vi "S4GUI.vi"(7 "Tab ObsEng":enum32{"Obs", "CCD modes", "Eng"}(tab)) -> ()   [LabVIEW 2018] (continued)
        n4535 = call "Write WPSEL.vi"("error in (no error)"=w10848, "Opt_Selector.lvclass"=w10850, "Instrument in"=w10849) -> ("error out"=w10845:errorcluster, "Instrument out"=w10847:refnum<class "Instrument.lvclass">)  [unwired: 7 in]
        n4536 = call "Write Instrument.lvclass.vi"("error in (no error)"=w10845, "Instrument.lvclass"=w10847, "S4ACS_GUI in"=w10846) -> ("error out"=w10844:errorcluster, "S4ACS_GUI out"=w10843:refnum<class "S4GUI.lvclass">)  [unwired: 7 in]
      }
      event "GMIR_target": Value Change {
        n4537 = event-data() -> ("NewVal"=w10872:dbl)  [unwired: 1 in, 3 out]
        n4538 = call "Read Instrument.lvclass.vi"("error in (no error)"=w10876, "S4ACS_GUI in"=w10877) -> ("error out"=w10874:errorcluster, "Instrument.lvclass"=w10875:refnum<class "Instrument.lvclass">, "S4ACS_GUI out"=w10866:refnum<class "S4GUI.lvclass">)  [unwired: 7 in]
        n4539 = call "Read GMIR.vi"("error in (no error)"=w10874, "Instrument in"=w10875) -> ("error out"=w10871:errorcluster, "Opt_Continuous.lvclass"=w10873:refnum<class "Opt_Continuous.lvclass">, "Instrument out"=w10869:refnum<class "Instrument.lvclass">)  [unwired: 7 in]
        n4540 = call "Write target.vi"("error in (no error)"=w10871, "target"=w10872, "Optics in"=w10873) -> ("error out"=w10868:errorcluster, "Optics out"=w10870:refnum<class "Opt_Continuous.lvclass">)  [unwired: 7 in]
        n4541 = call "Write GMIR.vi"("error in (no error)"=w10868, "Opt_Continuous.lvclass"=w10870, "Instrument in"=w10869) -> ("error out"=w10865:errorcluster, "Instrument out"=w10867:refnum<class "Instrument.lvclass">)  [unwired: 7 in]
        n4542 = call "Write Instrument.lvclass.vi"("error in (no error)"=w10865, "Instrument.lvclass"=w10867, "S4ACS_GUI in"=w10866) -> ("error out"=w10864:errorcluster, "S4ACS_GUI out"=w10863:refnum<class "S4GUI.lvclass">)  [unwired: 7 in]
      }
      event "GMIR_set": Value Change {
        n4543 = event-data() -> ()  [unwired: 1 in, 4 out]
        n4544 = call "Read Instrument.lvclass.vi"("error in (no error)"=w10896, "S4ACS_GUI in"=w10897) -> ("error out"=w10894:errorcluster, "Instrument.lvclass"=w10895:refnum<class "Instrument.lvclass">, "S4ACS_GUI out"=w10883:refnum<class "S4GUI.lvclass">)  [unwired: 7 in]
        n4545 = call "Read GMIR.vi"("error in (no error)"=w10894, "Instrument in"=w10895) -> ("error out"=w10891:errorcluster, "Opt_Continuous.lvclass"=w10893:refnum<class "Opt_Continuous.lvclass">, "Instrument out"=w10885:refnum<class "Instrument.lvclass">)  [unwired: 7 in]
        n4546 = call-dynamic "Read State Machine.vi"("error in (no error)"=w10891, "Device in"=w10893) -> ("error out"=w10890:errorcluster, "State Machine.lvclass"=w10881:refnum<class "State Machine.lvclass">, "Device out"=w10887:refnum<class "Opt_Continuous.lvclass">)  [unwired: 7 in]
        n4547 = call "Next State.vi"("error in (no error)"=w10890, "New_State"=1, "State Machine in"=w10881) -> ("error out"=w10889:errorcluster, "State Machine out"=w10888:refnum<class "State Machine.lvclass">)  [unwired: 7 in]
        n4548 = call-dynamic "Write State Machine.vi"("error in (no error)"=w10889, "State Machine.lvclass"=w10888, "Device in"=w10887) -> ("error out"=w10884:errorcluster, "Device out"=w10886:refnum<class "Opt_Continuous.lvclass">)  [unwired: 7 in]
        n4549 = call "Write GMIR.vi"("error in (no error)"=w10884, "Opt_Continuous.lvclass"=w10886, "Instrument in"=w10885) -> ("error out"=w10878:errorcluster, "Instrument out"=w10879:refnum<class "Instrument.lvclass">)  [unwired: 7 in]
        n4550 = call "Write Instrument.lvclass.vi"("error in (no error)"=w10878, "Instrument.lvclass"=w10879, "S4ACS_GUI in"=w10883) -> ("error out"=w10882:errorcluster, "S4ACS_GUI out"=w10880:refnum<class "S4GUI.lvclass">)  [unwired: 7 in]
      }
      event "GMIR_stop": Value Change {
        n4551 = event-data() -> ()  [unwired: 1 in, 4 out]
        n4552 = call "Read Instrument.lvclass.vi"("error in (no error)"=w10916, "S4ACS_GUI in"=w10917) -> ("error out"=w10914:errorcluster, "Instrument.lvclass"=w10915:refnum<class "Instrument.lvclass">, "S4ACS_GUI out"=w10901:refnum<class "S4GUI.lvclass">)  [unwired: 7 in]
        n4553 = call "Read GMIR.vi"("error in (no error)"=w10914, "Instrument in"=w10915) -> ("error out"=w10910:errorcluster, "Opt_Continuous.lvclass"=w10913:refnum<class "Opt_Continuous.lvclass">, "Instrument out"=w10904:refnum<class "Instrument.lvclass">)  [unwired: 7 in]
        n4554 = call-dynamic "Read State Machine.vi"("error in (no error)"=w10910, "Device in"=w10913) -> ("error out"=w10909:errorcluster, "State Machine.lvclass"=w10912:refnum<class "State Machine.lvclass">, "Device out"=w10906:refnum<class "Opt_Continuous.lvclass">)  [unwired: 7 in]
        n4555 = call "Next State.vi"("error in (no error)"=w10909, "New_State"=10, "State Machine in"=w10912) -> ("error out"=w10908:errorcluster, "State Machine out"=w10907:refnum<class "State Machine.lvclass">)  [unwired: 7 in]
        n4556 = call-dynamic "Write State Machine.vi"("error in (no error)"=w10908, "State Machine.lvclass"=w10907, "Device in"=w10906) -> ("error out"=w10903:errorcluster, "Device out"=w10905:refnum<class "Opt_Continuous.lvclass">)  [unwired: 7 in]
        n4557 = call "Write GMIR.vi"("error in (no error)"=w10903, "Opt_Continuous.lvclass"=w10905, "Instrument in"=w10904) -> ("error out"=w10900:errorcluster, "Instrument out"=w10902:refnum<class "Instrument.lvclass">)  [unwired: 7 in]
        n4558 = call "Write Instrument.lvclass.vi"("error in (no error)"=w10900, "Instrument.lvclass"=w10902, "S4ACS_GUI in"=w10901) -> ("error out"=w10899:errorcluster, "S4ACS_GUI out"=w10898:refnum<class "S4GUI.lvclass">)  [unwired: 7 in]
      }
      event "GMIR_init": Value Change {
        n4559 = event-data() -> ()  [unwired: 1 in, 4 out]
        n4560 = call "Read Instrument.lvclass.vi"("error in (no error)"=w10936, "S4ACS_GUI in"=w10937) -> ("error out"=w10934:errorcluster, "Instrument.lvclass"=w10935:refnum<class "Instrument.lvclass">, "S4ACS_GUI out"=w10921:refnum<class "S4GUI.lvclass">)  [unwired: 7 in]
        n4561 = call "Read GMIR.vi"("error in (no error)"=w10934, "Instrument in"=w10935) -> ("error out"=w10930:errorcluster, "Opt_Continuous.lvclass"=w10933:refnum<class "Opt_Continuous.lvclass">, "Instrument out"=w10924:refnum<class "Instrument.lvclass">)  [unwired: 7 in]
        n4562 = call-dynamic "Read State Machine.vi"("error in (no error)"=w10930, "Device in"=w10933) -> ("error out"=w10929:errorcluster, "State Machine.lvclass"=w10932:refnum<class "State Machine.lvclass">, "Device out"=w10926:refnum<class "Opt_Continuous.lvclass">)  [unwired: 7 in]
        n4563 = call "Next State.vi"("error in (no error)"=w10929, "New_State"=30, "State Machine in"=w10932) -> ("error out"=w10928:errorcluster, "State Machine out"=w10927:refnum<class "State Machine.lvclass">)  [unwired: 7 in]
        n4564 = call-dynamic "Write State Machine.vi"("error in (no error)"=w10928, "State Machine.lvclass"=w10927, "Device in"=w10926) -> ("error out"=w10923:errorcluster, "Device out"=w10925:refnum<class "Opt_Continuous.lvclass">)  [unwired: 7 in]
        n4565 = call "Write GMIR.vi"("error in (no error)"=w10923, "Opt_Continuous.lvclass"=w10925, "Instrument in"=w10924) -> ("error out"=w10920:errorcluster, "Instrument out"=w10922:refnum<class "Instrument.lvclass">)  [unwired: 7 in]
        n4566 = call "Write Instrument.lvclass.vi"("error in (no error)"=w10920, "Instrument.lvclass"=w10922, "S4ACS_GUI in"=w10921) -> ("error out"=w10919:errorcluster, "S4ACS_GUI out"=w10918:refnum<class "S4GUI.lvclass">)  [unwired: 7 in]
      }
      event "GFOC_target": Value Change {
        n4567 = event-data() -> ("NewVal"=w10947:dbl)  [unwired: 1 in, 3 out]
        n4568 = call "Read Instrument.lvclass.vi"("error in (no error)"=w10951, "S4ACS_GUI in"=w10952) -> ("error out"=w10949:errorcluster, "Instrument.lvclass"=w10950:refnum<class "Instrument.lvclass">, "S4ACS_GUI out"=w10941:refnum<class "S4GUI.lvclass">)  [unwired: 7 in]
        n4569 = call "Read GFOC.vi"("error in (no error)"=w10949, "Instrument in"=w10950) -> ("error out"=w10946:errorcluster, "Opt_Continuous.lvclass"=w10948:refnum<class "Opt_Continuous.lvclass">, "Instrument out"=w10944:refnum<class "Instrument.lvclass">)  [unwired: 7 in]
        n4570 = call "Write target.vi"("error in (no error)"=w10946, "target"=w10947, "Optics in"=w10948) -> ("error out"=w10943:errorcluster, "Optics out"=w10945:refnum<class "Opt_Continuous.lvclass">)  [unwired: 7 in]
        n4571 = call "Write GFOC.vi"("error in (no error)"=w10943, "Opt_Continuous.lvclass"=w10945, "Instrument in"=w10944) -> ("error out"=w10940:errorcluster, "Instrument out"=w10942:refnum<class "Instrument.lvclass">)  [unwired: 7 in]
        n4572 = call "Write Instrument.lvclass.vi"("error in (no error)"=w10940, "Instrument.lvclass"=w10942, "S4ACS_GUI in"=w10941) -> ("error out"=w10939:errorcluster, "S4ACS_GUI out"=w10938:refnum<class "S4GUI.lvclass">)  [unwired: 7 in]
      }
      event "GFOC_set": Value Change {
        n4573 = event-data() -> ()  [unwired: 1 in, 4 out]
        n4574 = call "Read Instrument.lvclass.vi"("error in (no error)"=w10971, "S4ACS_GUI in"=w10972) -> ("error out"=w10969:errorcluster, "Instrument.lvclass"=w10970:refnum<class "Instrument.lvclass">, "S4ACS_GUI out"=w10957:refnum<class "S4GUI.lvclass">)  [unwired: 7 in]
        n4575 = call "Read GFOC.vi"("error in (no error)"=w10969, "Instrument in"=w10970) -> ("error out"=w10966:errorcluster, "Opt_Continuous.lvclass"=w10968:refnum<class "Opt_Continuous.lvclass">, "Instrument out"=w10960:refnum<class "Instrument.lvclass">)  [unwired: 7 in]
        n4576 = call-dynamic "Read State Machine.vi"("error in (no error)"=w10966, "Device in"=w10968) -> ("error out"=w10965:errorcluster, "State Machine.lvclass"=w10954:refnum<class "State Machine.lvclass">, "Device out"=w10962:refnum<class "Opt_Continuous.lvclass">)  [unwired: 7 in]
        n4577 = call "Next State.vi"("error in (no error)"=w10965, "New_State"=1, "State Machine in"=w10954) -> ("error out"=w10964:errorcluster, "State Machine out"=w10963:refnum<class "State Machine.lvclass">)  [unwired: 7 in]
        n4578 = call-dynamic "Write State Machine.vi"("error in (no error)"=w10964, "State Machine.lvclass"=w10963, "Device in"=w10962) -> ("error out"=w10959:errorcluster, "Device out"=w10961:refnum<class "Opt_Continuous.lvclass">)  [unwired: 7 in]
        n4579 = call "Write GFOC.vi"("error in (no error)"=w10959, "Opt_Continuous.lvclass"=w10961, "Instrument in"=w10960) -> ("error out"=w10956:errorcluster, "Instrument out"=w10958:refnum<class "Instrument.lvclass">)  [unwired: 7 in]
        n4580 = call "Write Instrument.lvclass.vi"("error in (no error)"=w10956, "Instrument.lvclass"=w10958, "S4ACS_GUI in"=w10957) -> ("error out"=w10955:errorcluster, "S4ACS_GUI out"=w10953:refnum<class "S4GUI.lvclass">)  [unwired: 7 in]
      }
      event "GFOC_stop": Value Change {
        n4581 = event-data() -> ()  [unwired: 1 in, 4 out]
        n4582 = call "Read Instrument.lvclass.vi"("error in (no error)"=w10991, "S4ACS_GUI in"=w10992) -> ("error out"=w10989:errorcluster, "Instrument.lvclass"=w10990:refnum<class "Instrument.lvclass">, "S4ACS_GUI out"=w10976:refnum<class "S4GUI.lvclass">)  [unwired: 7 in]
        n4583 = call "Read GFOC.vi"("error in (no error)"=w10989, "Instrument in"=w10990) -> ("error out"=w10985:errorcluster, "Opt_Continuous.lvclass"=w10988:refnum<class "Opt_Continuous.lvclass">, "Instrument out"=w10979:refnum<class "Instrument.lvclass">)  [unwired: 7 in]
        n4584 = call-dynamic "Read State Machine.vi"("error in (no error)"=w10985, "Device in"=w10988) -> ("error out"=w10984:errorcluster, "State Machine.lvclass"=w10987:refnum<class "State Machine.lvclass">, "Device out"=w10981:refnum<class "Opt_Continuous.lvclass">)  [unwired: 7 in]
        n4585 = call "Next State.vi"("error in (no error)"=w10984, "New_State"=10, "State Machine in"=w10987) -> ("error out"=w10983:errorcluster, "State Machine out"=w10982:refnum<class "State Machine.lvclass">)  [unwired: 7 in]
        n4586 = call-dynamic "Write State Machine.vi"("error in (no error)"=w10983, "State Machine.lvclass"=w10982, "Device in"=w10981) -> ("error out"=w10978:errorcluster, "Device out"=w10980:refnum<class "Opt_Continuous.lvclass">)  [unwired: 7 in]
        n4587 = call "Write GFOC.vi"("error in (no error)"=w10978, "Opt_Continuous.lvclass"=w10980, "Instrument in"=w10979) -> ("error out"=w10975:errorcluster, "Instrument out"=w10977:refnum<class "Instrument.lvclass">)  [unwired: 7 in]
        n4588 = call "Write Instrument.lvclass.vi"("error in (no error)"=w10975, "Instrument.lvclass"=w10977, "S4ACS_GUI in"=w10976) -> ("error out"=w10974:errorcluster, "S4ACS_GUI out"=w10973:refnum<class "S4GUI.lvclass">)  [unwired: 7 in]
      }
      event "GFOC_init": Value Change {
        n4589 = event-data() -> ()  [unwired: 1 in, 4 out]
        n4590 = call "Read Instrument.lvclass.vi"("error in (no error)"=w11011, "S4ACS_GUI in"=w11012) -> ("error out"=w11009:errorcluster, "Instrument.lvclass"=w11010:refnum<class "Instrument.lvclass">, "S4ACS_GUI out"=w10996:refnum<class "S4GUI.lvclass">)  [unwired: 7 in]
        n4591 = call "Read GFOC.vi"("error in (no error)"=w11009, "Instrument in"=w11010) -> ("error out"=w11005:errorcluster, "Opt_Continuous.lvclass"=w11008:refnum<class "Opt_Continuous.lvclass">, "Instrument out"=w10999:refnum<class "Instrument.lvclass">)  [unwired: 7 in]
        n4592 = call-dynamic "Read State Machine.vi"("error in (no error)"=w11005, "Device in"=w11008) -> ("error out"=w11004:errorcluster, "State Machine.lvclass"=w11007:refnum<class "State Machine.lvclass">, "Device out"=w11001:refnum<class "Opt_Continuous.lvclass">)  [unwired: 7 in]
        n4593 = call "Next State.vi"("error in (no error)"=w11004, "New_State"=30, "State Machine in"=w11007) -> ("error out"=w11003:errorcluster, "State Machine out"=w11002:refnum<class "State Machine.lvclass">)  [unwired: 7 in]
        n4594 = call-dynamic "Write State Machine.vi"("error in (no error)"=w11003, "State Machine.lvclass"=w11002, "Device in"=w11001) -> ("error out"=w10998:errorcluster, "Device out"=w11000:refnum<class "Opt_Continuous.lvclass">)  [unwired: 7 in]
        n4595 = call "Write GFOC.vi"("error in (no error)"=w10998, "Opt_Continuous.lvclass"=w11000, "Instrument in"=w10999) -> ("error out"=w10995:errorcluster, "Instrument out"=w10997:refnum<class "Instrument.lvclass">)  [unwired: 7 in]
        n4596 = call "Write Instrument.lvclass.vi"("error in (no error)"=w10995, "Instrument.lvclass"=w10997, "S4ACS_GUI in"=w10996) -> ("error out"=w10994:errorcluster, "S4ACS_GUI out"=w10993:refnum<class "S4GUI.lvclass">)  [unwired: 7 in]
      }
      event "CALW_target": Value Change {
        n4597 = event-data() -> ("NewVal"=w11022:dbl)  [unwired: 1 in, 3 out]
        n4598 = call "Read Instrument.lvclass.vi"("error in (no error)"=w11026, "S4ACS_GUI in"=w11027) -> ("error out"=w11024:errorcluster, "Instrument.lvclass"=w11025:refnum<class "Instrument.lvclass">, "S4ACS_GUI out"=w11016:refnum<class "S4GUI.lvclass">)  [unwired: 7 in]
        n4599 = call "Read CALW.vi"("error in (no error)"=w11024, "Instrument in"=w11025) -> ("error out"=w11021:errorcluster, "Opt_Selector.lvclass"=w11023:refnum<class "Opt_Selector.lvclass">, "Instrument out"=w11019:refnum<class "Instrument.lvclass">)  [unwired: 7 in]
        n4600 = call "Write target.vi"("error in (no error)"=w11021, "target"=w11022, "Optics in"=w11023) -> ("error out"=w11018:errorcluster, "Optics out"=w11020:refnum<class "Opt_Selector.lvclass">)  [unwired: 7 in]
        n4601 = call "Write CALW.vi"("error in (no error)"=w11018, "Opt_Selector.lvclass"=w11020, "Instrument in"=w11019) -> ("error out"=w11015:errorcluster, "Instrument out"=w11017:refnum<class "Instrument.lvclass">)  [unwired: 7 in]
        n4602 = call "Write Instrument.lvclass.vi"("error in (no error)"=w11015, "Instrument.lvclass"=w11017, "S4ACS_GUI in"=w11016) -> ("error out"=w11014:errorcluster, "S4ACS_GUI out"=w11013:refnum<class "S4GUI.lvclass">)  [unwired: 7 in]
      }
      event "CALW_set": Value Change {
        n4603 = event-data() -> ()  [unwired: 1 in, 4 out]
        n4604 = call "Read Instrument.lvclass.vi"("error in (no error)"=w11046, "S4ACS_GUI in"=w11047) -> ("error out"=w11044:errorcluster, "Instrument.lvclass"=w11045:refnum<class "Instrument.lvclass">, "S4ACS_GUI out"=w11032:refnum<class "S4GUI.lvclass">)  [unwired: 7 in]
        n4605 = call "Read CALW.vi"("error in (no error)"=w11044, "Instrument in"=w11045) -> ("error out"=w11041:errorcluster, "Opt_Selector.lvclass"=w11043:refnum<class "Opt_Selector.lvclass">, "Instrument out"=w11035:refnum<class "Instrument.lvclass">)  [unwired: 7 in]
        n4606 = call-dynamic "Read State Machine.vi"("error in (no error)"=w11041, "Device in"=w11043) -> ("error out"=w11040:errorcluster, "State Machine.lvclass"=w11029:refnum<class "State Machine.lvclass">, "Device out"=w11037:refnum<class "Opt_Selector.lvclass">)  [unwired: 7 in]
        n4607 = call "Next State.vi"("error in (no error)"=w11040, "New_State"=1, "State Machine in"=w11029) -> ("error out"=w11039:errorcluster, "State Machine out"=w11038:refnum<class "State Machine.lvclass">)  [unwired: 7 in]
        n4608 = call-dynamic "Write State Machine.vi"("error in (no error)"=w11039, "State Machine.lvclass"=w11038, "Device in"=w11037) -> ("error out"=w11034:errorcluster, "Device out"=w11036:refnum<class "Opt_Selector.lvclass">)  [unwired: 7 in]
        n4609 = call "Write CALW.vi"("error in (no error)"=w11034, "Opt_Selector.lvclass"=w11036, "Instrument in"=w11035) -> ("error out"=w11031:errorcluster, "Instrument out"=w11033:refnum<class "Instrument.lvclass">)  [unwired: 7 in]
        n4610 = call "Write Instrument.lvclass.vi"("error in (no error)"=w11031, "Instrument.lvclass"=w11033, "S4ACS_GUI in"=w11032) -> ("error out"=w11030:errorcluster, "S4ACS_GUI out"=w11028:refnum<class "S4GUI.lvclass">)  [unwired: 7 in]
      }
      event "CALW_stop": Value Change {
        n4611 = event-data() -> ()  [unwired: 1 in, 4 out]
        n4612 = call "Read Instrument.lvclass.vi"("error in (no error)"=w11066, "S4ACS_GUI in"=w11067) -> ("error out"=w11064:errorcluster, "Instrument.lvclass"=w11065:refnum<class "Instrument.lvclass">, "S4ACS_GUI out"=w11051:refnum<class "S4GUI.lvclass">)  [unwired: 7 in]
        n4613 = call "Read CALW.vi"("error in (no error)"=w11064, "Instrument in"=w11065) -> ("error out"=w11060:errorcluster, "Opt_Selector.lvclass"=w11063:refnum<class "Opt_Selector.lvclass">, "Instrument out"=w11054:refnum<class "Instrument.lvclass">)  [unwired: 7 in]
        n4614 = call-dynamic "Read State Machine.vi"("error in (no error)"=w11060, "Device in"=w11063) -> ("error out"=w11059:errorcluster, "State Machine.lvclass"=w11062:refnum<class "State Machine.lvclass">, "Device out"=w11056:refnum<class "Opt_Selector.lvclass">)  [unwired: 7 in]
        n4615 = call "Next State.vi"("error in (no error)"=w11059, "New_State"=10, "State Machine in"=w11062) -> ("error out"=w11058:errorcluster, "State Machine out"=w11057:refnum<class "State Machine.lvclass">)  [unwired: 7 in]
        n4616 = call-dynamic "Write State Machine.vi"("error in (no error)"=w11058, "State Machine.lvclass"=w11057, "Device in"=w11056) -> ("error out"=w11053:errorcluster, "Device out"=w11055:refnum<class "Opt_Selector.lvclass">)  [unwired: 7 in]
        n4617 = call "Write CALW.vi"("error in (no error)"=w11053, "Opt_Selector.lvclass"=w11055, "Instrument in"=w11054) -> ("error out"=w11050:errorcluster, "Instrument out"=w11052:refnum<class "Instrument.lvclass">)  [unwired: 7 in]
        n4618 = call "Write Instrument.lvclass.vi"("error in (no error)"=w11050, "Instrument.lvclass"=w11052, "S4ACS_GUI in"=w11051) -> ("error out"=w11049:errorcluster, "S4ACS_GUI out"=w11048:refnum<class "S4GUI.lvclass">)  [unwired: 7 in]
      }
      event "CALW_init": Value Change {
        n4619 = event-data() -> ()  [unwired: 1 in, 4 out]
        n4620 = call "Read Instrument.lvclass.vi"("error in (no error)"=w11086, "S4ACS_GUI in"=w11087) -> ("error out"=w11084:errorcluster, "Instrument.lvclass"=w11085:refnum<class "Instrument.lvclass">, "S4ACS_GUI out"=w11071:refnum<class "S4GUI.lvclass">)  [unwired: 7 in]
        n4621 = call "Read CALW.vi"("error in (no error)"=w11084, "Instrument in"=w11085) -> ("error out"=w11080:errorcluster, "Opt_Selector.lvclass"=w11083:refnum<class "Opt_Selector.lvclass">, "Instrument out"=w11074:refnum<class "Instrument.lvclass">)  [unwired: 7 in]
        n4622 = call-dynamic "Read State Machine.vi"("error in (no error)"=w11080, "Device in"=w11083) -> ("error out"=w11079:errorcluster, "State Machine.lvclass"=w11082:refnum<class "State Machine.lvclass">, "Device out"=w11076:refnum<class "Opt_Selector.lvclass">)  [unwired: 7 in]
        n4623 = call "Next State.vi"("error in (no error)"=w11079, "New_State"=30, "State Machine in"=w11082) -> ("error out"=w11078:errorcluster, "State Machine out"=w11077:refnum<class "State Machine.lvclass">)  [unwired: 7 in]
        n4624 = call-dynamic "Write State Machine.vi"("error in (no error)"=w11078, "State Machine.lvclass"=w11077, "Device in"=w11076) -> ("error out"=w11073:errorcluster, "Device out"=w11075:refnum<class "Opt_Selector.lvclass">)  [unwired: 7 in]
        n4625 = call "Write CALW.vi"("error in (no error)"=w11073, "Opt_Selector.lvclass"=w11075, "Instrument in"=w11074) -> ("error out"=w11070:errorcluster, "Instrument out"=w11072:refnum<class "Instrument.lvclass">)  [unwired: 7 in]
        n4626 = call "Write Instrument.lvclass.vi"("error in (no error)"=w11070, "Instrument.lvclass"=w11072, "S4ACS_GUI in"=w11071) -> ("error out"=w11069:errorcluster, "S4ACS_GUI out"=w11068:refnum<class "S4GUI.lvclass">)  [unwired: 7 in]
      }
      event "ASEL_target": Value Change {
        n4627 = event-data() -> ("NewVal"=w11097:dbl)  [unwired: 1 in, 3 out]
        n4628 = call "Read Instrument.lvclass.vi"("error in (no error)"=w11101, "S4ACS_GUI in"=w11102) -> ("error out"=w11099:errorcluster, "Instrument.lvclass"=w11100:refnum<class "Instrument.lvclass">, "S4ACS_GUI out"=w11091:refnum<class "S4GUI.lvclass">)  [unwired: 7 in]
        n4629 = call "Read ASEL.vi"("error in (no error)"=w11099, "Instrument in"=w11100) -> ("error out"=w11096:errorcluster, "Opt_Selector.lvclass"=w11098:refnum<class "Opt_Selector.lvclass">, "Instrument out"=w11094:refnum<class "Instrument.lvclass">)  [unwired: 7 in]
        n4630 = call "Write target.vi"("error in (no error)"=w11096, "target"=w11097, "Optics in"=w11098) -> ("error out"=w11093:errorcluster, "Optics out"=w11095:refnum<class "Opt_Selector.lvclass">)  [unwired: 7 in]
        n4631 = call "Write ASEL.vi"("error in (no error)"=w11093, "Opt_Selector.lvclass"=w11095, "Instrument in"=w11094) -> ("error out"=w11090:errorcluster, "Instrument out"=w11092:refnum<class "Instrument.lvclass">)  [unwired: 7 in]
        n4632 = call "Write Instrument.lvclass.vi"("error in (no error)"=w11090, "Instrument.lvclass"=w11092, "S4ACS_GUI in"=w11091) -> ("error out"=w11089:errorcluster, "S4ACS_GUI out"=w11088:refnum<class "S4GUI.lvclass">)  [unwired: 7 in]
      }
      event "ASEL_set": Value Change {
        n4633 = event-data() -> ()  [unwired: 1 in, 4 out]
        n4634 = call "Read Instrument.lvclass.vi"("error in (no error)"=w11121, "S4ACS_GUI in"=w11122) -> ("error out"=w11119:errorcluster, "Instrument.lvclass"=w11120:refnum<class "Instrument.lvclass">, "S4ACS_GUI out"=w11107:refnum<class "S4GUI.lvclass">)  [unwired: 7 in]
        n4635 = call "Read ASEL.vi"("error in (no error)"=w11119, "Instrument in"=w11120) -> ("error out"=w11116:errorcluster, "Opt_Selector.lvclass"=w11118:refnum<class "Opt_Selector.lvclass">, "Instrument out"=w11110:refnum<class "Instrument.lvclass">)  [unwired: 7 in]
        n4636 = call-dynamic "Read State Machine.vi"("error in (no error)"=w11116, "Device in"=w11118) -> ("error out"=w11115:errorcluster, "State Machine.lvclass"=w11104:refnum<class "State Machine.lvclass">, "Device out"=w11112:refnum<class "Opt_Selector.lvclass">)  [unwired: 7 in]
        n4637 = call "Next State.vi"("error in (no error)"=w11115, "New_State"=1, "State Machine in"=w11104) -> ("error out"=w11114:errorcluster, "State Machine out"=w11113:refnum<class "State Machine.lvclass">)  [unwired: 7 in]
        n4638 = call-dynamic "Write State Machine.vi"("error in (no error)"=w11114, "State Machine.lvclass"=w11113, "Device in"=w11112) -> ("error out"=w11109:errorcluster, "Device out"=w11111:refnum<class "Opt_Selector.lvclass">)  [unwired: 7 in]
        n4639 = call "Write ASEL.vi"("error in (no error)"=w11109, "Opt_Selector.lvclass"=w11111, "Instrument in"=w11110) -> ("error out"=w11106:errorcluster, "Instrument out"=w11108:refnum<class "Instrument.lvclass">)  [unwired: 7 in]
        n4640 = call "Write Instrument.lvclass.vi"("error in (no error)"=w11106, "Instrument.lvclass"=w11108, "S4ACS_GUI in"=w11107) -> ("error out"=w11105:errorcluster, "S4ACS_GUI out"=w11103:refnum<class "S4GUI.lvclass">)  [unwired: 7 in]
      }
      event "ASEL_stop": Value Change {
        n4641 = event-data() -> ()  [unwired: 1 in, 4 out]
        n4642 = call "Read Instrument.lvclass.vi"("error in (no error)"=w11141, "S4ACS_GUI in"=w11142) -> ("error out"=w11139:errorcluster, "Instrument.lvclass"=w11140:refnum<class "Instrument.lvclass">, "S4ACS_GUI out"=w11126:refnum<class "S4GUI.lvclass">)  [unwired: 7 in]
        n4643 = call "Read ASEL.vi"("error in (no error)"=w11139, "Instrument in"=w11140) -> ("error out"=w11135:errorcluster, "Opt_Selector.lvclass"=w11138:refnum<class "Opt_Selector.lvclass">, "Instrument out"=w11129:refnum<class "Instrument.lvclass">)  [unwired: 7 in]
        n4644 = call-dynamic "Read State Machine.vi"("error in (no error)"=w11135, "Device in"=w11138) -> ("error out"=w11134:errorcluster, "State Machine.lvclass"=w11137:refnum<class "State Machine.lvclass">, "Device out"=w11131:refnum<class "Opt_Selector.lvclass">)  [unwired: 7 in]
        n4645 = call "Next State.vi"("error in (no error)"=w11134, "New_State"=10, "State Machine in"=w11137) -> ("error out"=w11133:errorcluster, "State Machine out"=w11132:refnum<class "State Machine.lvclass">)  [unwired: 7 in]
        n4646 = call-dynamic "Write State Machine.vi"("error in (no error)"=w11133, "State Machine.lvclass"=w11132, "Device in"=w11131) -> ("error out"=w11128:errorcluster, "Device out"=w11130:refnum<class "Opt_Selector.lvclass">)  [unwired: 7 in]
        n4647 = call "Write ASEL.vi"("error in (no error)"=w11128, "Opt_Selector.lvclass"=w11130, "Instrument in"=w11129) -> ("error out"=w11125:errorcluster, "Instrument out"=w11127:refnum<class "Instrument.lvclass">)  [unwired: 7 in]
        n4648 = call "Write Instrument.lvclass.vi"("error in (no error)"=w11125, "Instrument.lvclass"=w11127, "S4ACS_GUI in"=w11126) -> ("error out"=w11124:errorcluster, "S4ACS_GUI out"=w11123:refnum<class "S4GUI.lvclass">)  [unwired: 7 in]
      }
      event "ASEL_init": Value Change {
        n4649 = event-data() -> ()  [unwired: 1 in, 4 out]
        n4650 = call "Read Instrument.lvclass.vi"("error in (no error)"=w11161, "S4ACS_GUI in"=w11162) -> ("error out"=w11159:errorcluster, "Instrument.lvclass"=w11160:refnum<class "Instrument.lvclass">, "S4ACS_GUI out"=w11146:refnum<class "S4GUI.lvclass">)  [unwired: 7 in]
        n4651 = call "Read ASEL.vi"("error in (no error)"=w11159, "Instrument in"=w11160) -> ("error out"=w11155:errorcluster, "Opt_Selector.lvclass"=w11158:refnum<class "Opt_Selector.lvclass">, "Instrument out"=w11149:refnum<class "Instrument.lvclass">)  [unwired: 7 in]
        n4652 = call-dynamic "Read State Machine.vi"("error in (no error)"=w11155, "Device in"=w11158) -> ("error out"=w11154:errorcluster, "State Machine.lvclass"=w11157:refnum<class "State Machine.lvclass">, "Device out"=w11151:refnum<class "Opt_Selector.lvclass">)  [unwired: 7 in]
        n4653 = call "Next State.vi"("error in (no error)"=w11154, "New_State"=30, "State Machine in"=w11157) -> ("error out"=w11153:errorcluster, "State Machine out"=w11152:refnum<class "State Machine.lvclass">)  [unwired: 7 in]
        n4654 = call-dynamic "Write State Machine.vi"("error in (no error)"=w11153, "State Machine.lvclass"=w11152, "Device in"=w11151) -> ("error out"=w11148:errorcluster, "Device out"=w11150:refnum<class "Opt_Selector.lvclass">)  [unwired: 7 in]
        n4655 = call "Write ASEL.vi"("error in (no error)"=w11148, "Opt_Selector.lvclass"=w11150, "Instrument in"=w11149) -> ("error out"=w11145:errorcluster, "Instrument out"=w11147:refnum<class "Instrument.lvclass">)  [unwired: 7 in]
        n4656 = call "Write Instrument.lvclass.vi"("error in (no error)"=w11145, "Instrument.lvclass"=w11147, "S4ACS_GUI in"=w11146) -> ("error out"=w11144:errorcluster, "S4ACS_GUI out"=w11143:refnum<class "S4GUI.lvclass">)  [unwired: 7 in]
      }
    }
    n4657 = Unbundle By Name(w71) -> ("status"=w70:bool)
    n4658 = flat-sequence {
      tunnel: w85 -> [w102]
      tunnel: w83 -> [w100]
      tunnel: [w102] -> w82
      tunnel: [w98] -> w81
      tunnel: [w97] -> w80
      tunnel: [w105] -> w84
      tunnel: w82 -> [w105]
      tunnel: w81 -> [w104]
      tunnel: w80 -> [w103]
      frame #0 {
        n4659 = Tick Count (ms)() -> (millisecond timer value=w101:u32)
        n4660 = local read "loop max(ms)"() -> (w96:u32)
        n4661 = Subtract(x=w101, y=w100) -> (x-y=w98:u32)
        n4662 = Greater?(x=w98, y=w96) -> (0:w99:bool)
        n4663 = Select(t=w98, s=w99, f=w96) -> (s? t:f=w97:u32)
      }
      frame #1 {
        "loop time(ms)" <- w104
        "loop max(ms)" <- w103
      }
    }
    n4664 = Or(x=w70, y=w69) -> (x .or. y?=w68:bool)
  }
  "error out 9" <- w20
  n4665 = while {
    tunnel: w5 -> [_]
    stop <- FALSE stop-if-true
    n4666 = call "ZeroMQ_ACS1.vi"() -> ()  [unwired: 12 in]
    n4667 = call "ZeroMQ_ACS2.vi"() -> ()  [unwired: 12 in]
    n4668 = call "ZeroMQ_ACS3.vi"() -> ()  [unwired: 12 in]
    n4669 = call "ZeroMQ_ACS4.vi"() -> ()  [unwired: 12 in]
    n4670 = disable-structure shown="Enabled" {
      frame Disabled {
        n4671 = call "ZeroMQ_FOC.vi"() -> ()  [unwired: 12 in]
      }
      frame Enabled {
        n4672 = call "ZeroMQ_FOC_REQREP.vi"() -> ()  [unwired: 12 in]
      }
    }
    n4673 = call "ZeroMQ_WSTA.vi"() -> ()  [unwired: 12 in]
    n4674 = call "ZeroMQ_TCS.vi"() -> ()  [unwired: 12 in]
    n4675 = call "ZeroMQ_S4ICS.vi"() -> ()  [unwired: 12 in]
    n4676 = call "ZeroMQ_SUBGS.vi"() -> ()  [unwired: 12 in]
    n4677 = call "StreamTransmitSyncBox.vi"() -> ()  [unwired: 12 in]
    n4678 = call "StreamReceiveSyncBox.vi"() -> ()  [unwired: 12 in]
    n4679 = call "ZeroMQ_PUB.vi"() -> ()  [unwired: 12 in]
  }
  n4680 = stacked-sequence "INTERFACE" {
    frame #0 {
    }
    frame #1 {
    }
    frame #2 {
    }
    frame #3 {
    }
    frame #4 {
    }
    frame #5 {
    }
    frame #6 {
    }
  }
  n4681 = call-dynamic "End.vi"("S4ACS_GUI in"=w44) -> ("error out"=w8:errorcluster)  [unwired: 9 in, 1 out]
  n4682 = flat-sequence {
    tunnel: [w11165] -> w2
    tunnel: w8 -> [w11167]
    tunnel: [w11173] -> w7
    tunnel: w2 -> [w11173]
    frame #0 {
      w11171 = FALSE
      # "Apaga todos os leds, habilita Tab ObsEng."
      n4683 = property on="Tab ObsEng" class="TabCtl (strict)"("Tabs Visible?"=TRUE) -> ()  [unwired: 2 in, 2 out]
      n4684 = property on="Channel 4" class="Bool (strict)"("Value"=w11171) -> ()  [unwired: 2 in, 2 out]
      n4685 = property on="Channel 3" class="Bool (strict)"("Value"=w11171) -> ()  [unwired: 2 in, 2 out]
      n4686 = property on="Channel 2" class="Bool (strict)"("Value"=w11171) -> ()  [unwired: 2 in, 2 out]
      n4687 = property on="Channel 1" class="Bool (strict)"("Value"=w11171) -> ()  [unwired: 2 in, 2 out]
      n4688 = property on="S4ICSoft" class="Bool (strict)"("Value"=w11171) -> ()  [unwired: 2 in, 2 out]
      n4689 = call <vilib>:"Clear Errors.vi"("error in (no error)"=w11167) -> ("error out"=w11164:errorcluster)  [unwired: 5 in, 1 out]
      n4690 = property on="TCSPD" class="Bool (strict)"("Value"=w11171) -> ()  [unwired: 2 in, 2 out]
      n4691 = property on="Focus 160" class="Bool (strict)"("Value"=w11171) -> ()  [unwired: 2 in, 2 out]
      n4692 = property on="Weather" class="Bool (strict)"("Value"=w11171) -> ()  [unwired: 2 in, 2 out]
      n4693 = property on="GUIDER" class="Bool (strict)"("Value"=w11171) -> ()  [unwired: 2 in, 2 out]
      n4694 = disable-structure shown="Disabled" {
        frame Disabled {
          n4695 = local write "Last Error"("" ("Last Error")) -> ()
        }
        frame Enabled {
        }
      }
      n4696 = property on="Last Error" class="Str"(error in=w11164, "Text.BG Color"=u32 13816530 ("Color Box"), "Caption.FontBold"=FALSE ("Caption.Font:Bold")) -> (error out=w11166:errorcluster)  [unwired: 1 in, 1 out]
      n4697 = call <vilib>:"Clear Errors.vi"("error in (no error)"=w11166) -> ("error out"=w11165:errorcluster)  [unwired: 5 in, 1 out]
    }
    frame #1 {
      n4698 = Stop() -> ()  [unwired: 1 in]
    }
  }
  "error out" <- w7
  "GUI version" <- w11
